vi "Verify Message Command.vi"(5 "Instruction ID":i32, 6 "Cmd Address":u16 format="%04x", 7 "Target IC (1-8)":u8, 8 "error in (no error)":errorcluster, 9 "Transmit?":bool, 10 "RT-RT?":bool, 11 "BC Major Frame in":refnum<class "BC Major Frame.lvclass">) -> (0 "error out":errorcluster, 3 "BC Major Frame out":refnum<class "BC Major Frame.lvclass">, 4 "Post-Data Address":u16 format="%04x")   [LabVIEW 2016, in "BC Major Frame.lvclass"]
uses:
  BC Major Frame.lvclass
  PPLs/FPGA Interface.lvlibp/FPGA Interface/FPGA Interface.lvclass
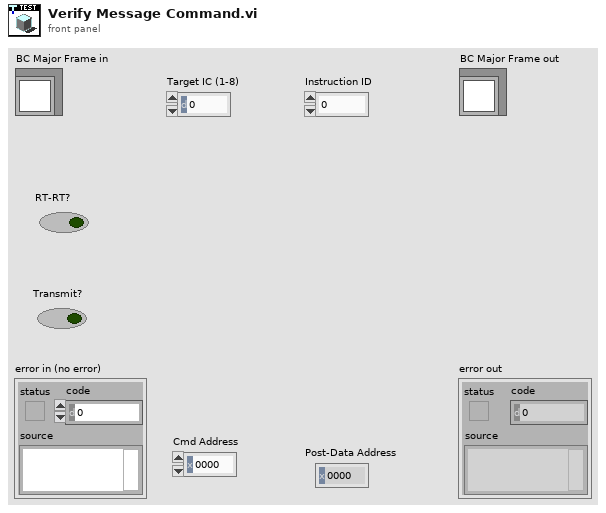
[diagram p1: front panel]
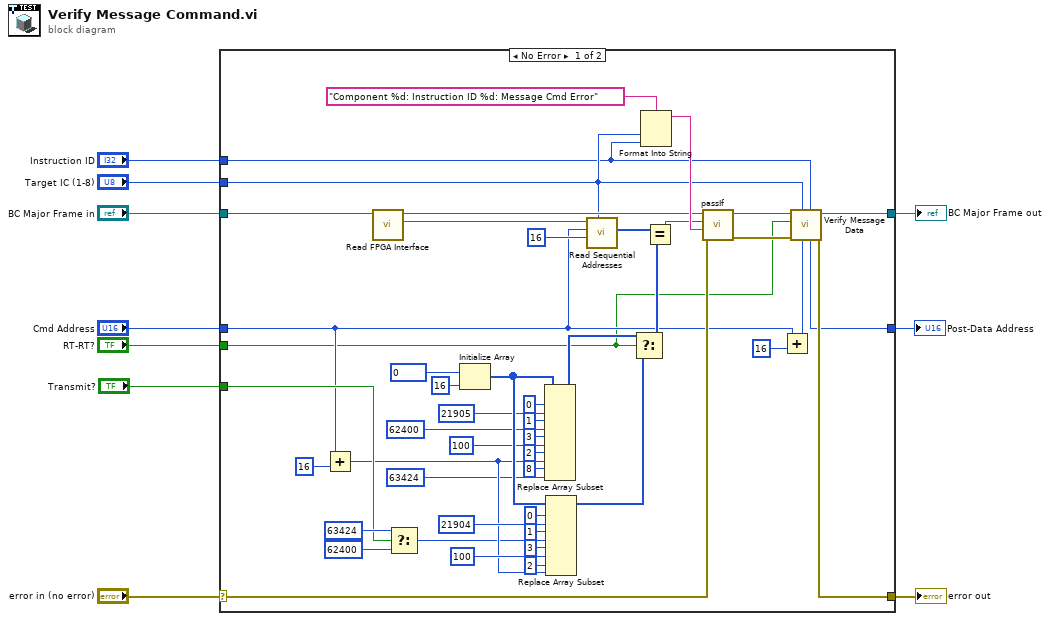
[diagram p0: block diagram]
diagram:
  n1 = case shown="No Error" "error in (no error)" {
    selector: "error in (no error)" -> [w55 w60]
    tunnel: [w42 w60] -> w9
    tunnel: [w11 w59] -> w7
    tunnel: "BC Major Frame in" -> [w49 w59]
    tunnel: "Instruction ID" -> [w13 _]
    tunnel: "Target IC (1-8)" -> [w14 _]
    tunnel: "Cmd Address" -> [w23 w58]
    tunnel: [w12 w58] -> w3
    tunnel: "RT-RT?" -> [w15 _]
    tunnel: "Transmit?" -> [w30 _]
    frame No Error {
      n2 = Add(x=w23, y=u16 16) -> (x+y=w20:u16)
      n3 = call-dynamic "Read FPGA Interface.vi"("1553 Test in"=w49) -> ("FPGA Interface"=w50:refnum<class "FPGA Interface.lvclass">, "1553 Test out"=w48:refnum<class "BC Major Frame.lvclass">)  [unwired: 8 in, 1 out]
      n4 = Select(t=u16 63424, s=w30, f=u16 62400) -> (s? t:f=w17:u16)
      n5 = Initialize Array(u16 0, 16 ("dimension size")) -> (w39:u16[])
      n6 = Replace Array Subset(array=w39, new element #1=u16 21905, index #1=0 ("index"), new element #2=u16 62400, index #2=1 ("index"), new element #3=u16 100 ("dimension size"), index #3=3 ("index"), new element #4=w20, index #4=2 ("index"), new element #5=u16 63424, index #5=8 ("index")) -> (w40:u16[])
      n7 = Replace Array Subset(array=w39, new element #1=u16 21904, index #1=0 ("index"), new element #2=w17, index #2=1 ("index"), new element #3=u16 100 ("new element/subarray"), index #3=3 ("index"), new element #4=w20, index #4=2 ("index")) -> (w34:u16[])
      n8 = call-dynamic "Read Sequential Addresses.vi"("Target IC (1-8)"=w14, "Addresses to Read"=u16 16, "Starting Address"=w23, "FPGA Interface in"=w50) -> ("Data"=w47:u16[])  [unwired: 6 in, 1 out]
      n9 = Select(t=w40, s=w15, f=w34) -> (s? t:f=w46:u16[])
      n10 = Format Into String(format string="Component %d: Instruction ID %d: Message Cmd Error" ("message (\"\")"), w14, w13) -> (resulting string=w57:string)  [unwired: 2 in, 1 out]
      n11 = Equal?(x=w47, y=w46) -> (x = y?=w45:bool)
      n12 = call-dynamic "passIf.vi"("error in (no error)"=w55, "message (\"\")"=w57, "pass"=w45, "TestCase in"=w48) -> ("error out"=w43:errorcluster, "TestCase out"=w44:refnum<class "BC Major Frame.lvclass">)  [unwired: 6 in]
      n13 = Add(x=w23, y=u16 16) -> (x+y=w41:u16)
      n14 = call-dynamic "Verify Message Data.vi"("Instruction ID"=w13, "Data Address"=w41, "Target IC (1-8)"=w14, "error in (no error)"=w43, "RT-RT?"=w15, "BC Major Frame in"=w44) -> ("error out"=w42:errorcluster, "BC Major Frame out"=w11:refnum<class "BC Major Frame.lvclass">, "Post-Data Address"=w12:u16)  [unwired: 3 in]
    }
    frame Error {
    }
  }
  "error out" <- w9
  "BC Major Frame out" <- w7
  "Post-Data Address" <- w3
